vi "SendMessage.vi"(8 "error in (no error)":errorcluster, 10 "data in":string, 11 "STOMP in":refnum<class "STOMP.lvclass">) -> (0 "error out":errorcluster, 3 "STOMP out":refnum<class "STOMP.lvclass">)   [LabVIEW 2017, in "LabVIEW STOMP.lvlib" / "STOMP.lvclass"]
uses:
  STOMP.lvclass
  STOMP.lvclass/STOMP.ctl
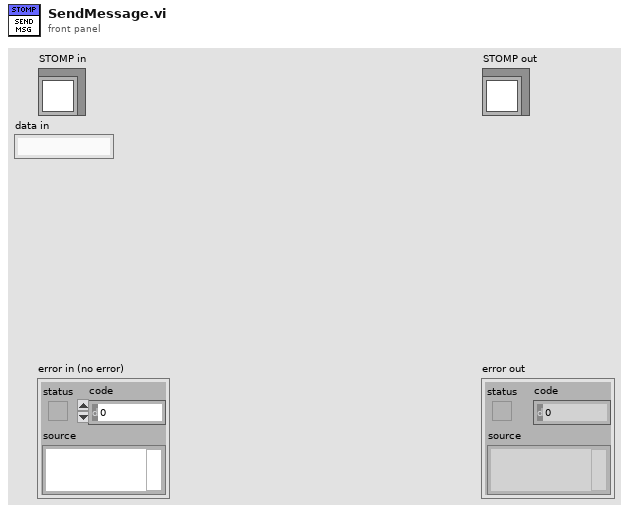
[diagram p1: front panel]
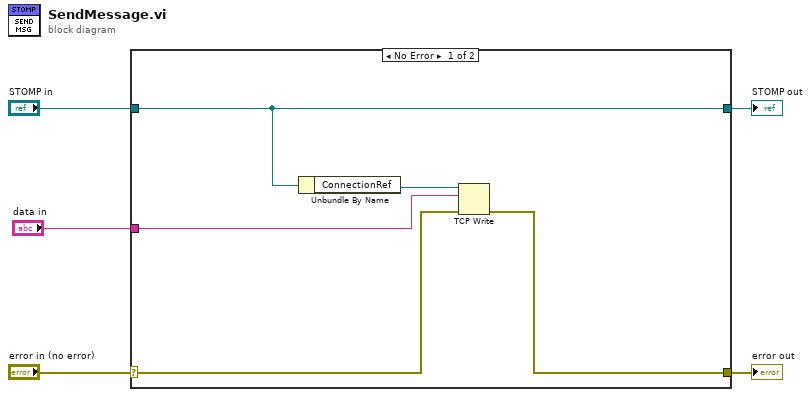
[diagram p0: block diagram]
diagram:
  n1 = case shown="No Error" "error in (no error)" {
    selector: "error in (no error)" -> [w7 w12]
    tunnel: [w6 w12] -> w4
    tunnel: [w10 w11] -> w2
    tunnel: "STOMP in" -> [w10 w11]
    tunnel: "data in" -> [w8 _]
    frame No Error {
      n2 = Unbundle By Name(w10) -> ("ConnectionRef"=w9:refnum<k5>)
      n3 = TCP Write(connection ID=w9, data in=w8, error in (no error)=w7) -> (error out=w6:errorcluster)  [unwired: 1 in, 2 out]
    }
    frame Error {
    }
  }
  "error out" <- w4
  "STOMP out" <- w2
